vi "Trigger Rolling Array - Constant (SubVI).vi"(0 "Waveform Input":waveform(dbl), 2 "Max Elapsed Build Time (ms)":dbl, 5 "Reset Timer":bool=TRUE) -> (16 "Waveform Array":T1(array[cluster]), 18 "Build Array Complete?":bool)   [LabVIEW 2009]
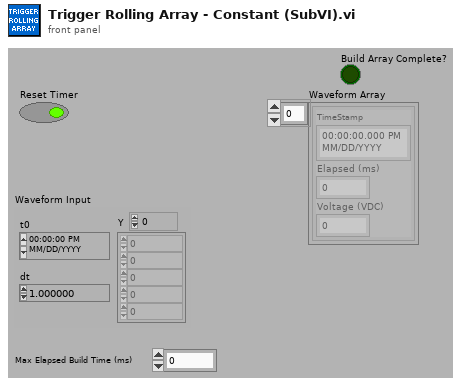
[diagram p1: front panel]
types:
  T1 = cluster{"TimeStamp":timestamp, "Elapsed (ms)":dbl, "Voltage (VDC)":dbl}[]
  T2 = cluster{"TimeStamp":timestamp, "Elapsed (ms)":dbl, "Voltage (VDC)":dbl}
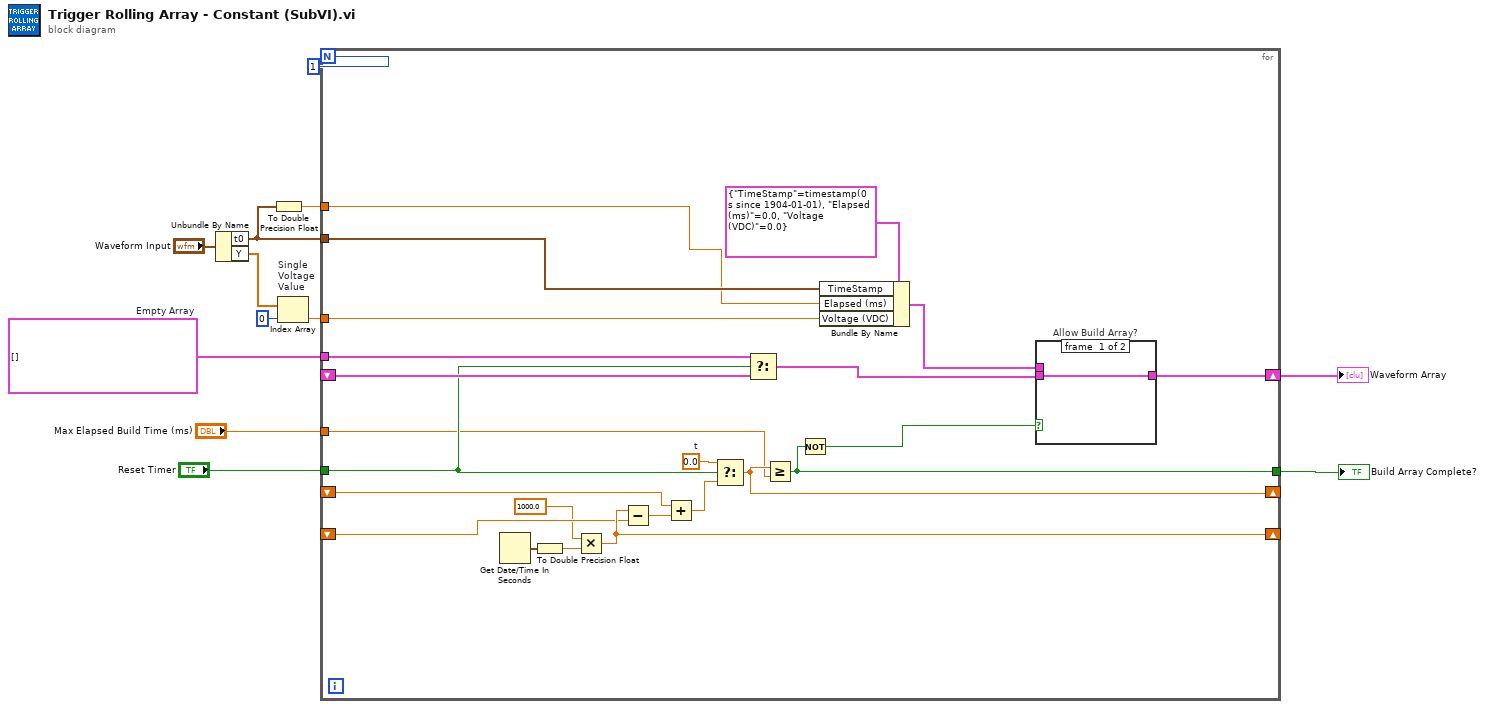
[diagram p0: block diagram]
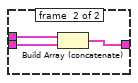
[diagram p2: hidden frame]
diagram:
  w7 = T1 []  # Empty Array
  n1 = Unbundle By Name("Waveform Input") -> ("t0"=w8:timestamp, "Y"=w5:dbl[])
  n2 = To Double Precision Float(number=w8) -> (double precision float=w9:dbl)
  n3 = Index Array "Single\nVoltage\nValue"(array=w5, index=0) -> (element=w6:dbl)
  n4 = for {
    N: 1 -> [_]
    tunnel: "Reset Timer" -> [w16]
    tunnel: w8 -> [w34]
    tunnel: w6 -> [w22]
    shift-right: [w20] -> w12
    shift-left: _ -> [w31]
    tunnel: w7 -> [w32]
    tunnel: w9 -> [w18]
    tunnel: "Max Elapsed Build Time (ms)" -> [w15]
    shift-right: [w27] -> _
    shift-left: _ -> [w26]
    shift-right: [w19] -> _
    shift-left: _ -> [w24]
    tunnel: [w14] -> w1
    w17 = 0.0  # t
    n5 = Get Date/Time In Seconds() -> (seconds since 1Jan1904=w30:timestamp)
    n6 = To Double Precision Float(number=w30) -> (double precision float=w25:dbl)
    n7 = Multiply(x=1000.0 ("y"), y=w25) -> (x*y=w27:dbl)
    n8 = Subtract(x=w27, y=w26) -> (x-y=w29:dbl)
    n9 = Add(x=w24, y=w29) -> (x+y=w28:dbl)
    n10 = Select(t=w17, s=w16, f=w28) -> (s? t:f=w19:dbl)
    n11 = Select(t=w32, s=w16, f=w31) -> (s? t:f=w21:T1)
    n12 = Greater Or Equal?(x=w19, y=w15) -> (x >= y?=w14:bool)
    n13 = Not(x=w14) -> (.not. x?=w13:bool)
    n14 = Bundle By Name(cluster=T2 {"TimeStamp"=timestamp(0 s since 1904-01-01), "Elapsed (ms)"=0.0, "Voltage (VDC)"=0.0}, "TimeStamp"=w34, "Elapsed (ms)"=w18, "Voltage (VDC)"=w22) -> (w33:T2)
    n15 = case "Allow Build Array?" shown="True" w13 {
      tunnel: w33 -> [_ w39]
      tunnel: [w36 w38] -> w20
      tunnel: w21 -> [w36 w37]
      frame #0 {
      }
      frame #1 {
        n16 = Build Array (concatenate)(w39, w37) -> (w38:T1)
      }
    }
  }
  "Waveform Array" <- w12
  "Build Array Complete?" <- w1
